vi "Double Array.vi"(8 "Error In":errorcluster) -> (0 "Error Out":errorcluster)   [LabVIEW 2017, in "Tests.lvlib" / "To Msgpack.lvlib"]
uses:
  To Msgpack.lvlib
  <vilib>/addons/_JKI Toolkits/Caraya/classes/Test/Test.lvclass
  src/LabPack/LabPack.lvlib
  <vilib>/addons/_JKI Toolkits/Caraya/classes/Assert/Assert.lvclass
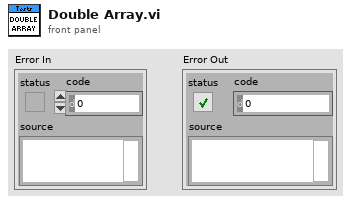
[diagram p1: front panel]
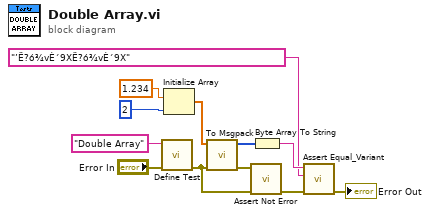
[diagram p0: block diagram]
diagram:
  n1 = call <vilib>:"Define Test.vi"("error in (no error)"="Error In", "Label (VI Title)"="Double Array") -> ("error out"=w8:errorcluster)  [unwired: 9 in]
  n2 = Initialize Array(1.234, 2 ("dimension size")) -> (w6:dbl[])
  n3 = call "To Msgpack.vi"("Error In"=w8, "Anything"=w6) -> ("Error Out"=w9:errorcluster, "Msgpack Data"=w3:u8[])  [unwired: 8 in]
  n4 = call <vilib>:"Assert Not Error.vi"("error in (no error)"=w8, "Not Error?"=w9) -> ("error out"=w10:errorcluster)  [unwired: 9 in]
  n5 = Byte Array To String(unsigned byte array=w3) -> (string=w2:string)
  n6 = call <vilib>:"Assert Equal_Variant.vi"("error in (no error)"=w10, "Y"="’Ë?ó¾vÈ´9XË?ó¾vÈ´9X" ("string"), "X"=w2) -> ("error out"=→"Error Out":errorcluster)  [unwired: 8 in]
